vi "MCA_OpenDialog.vi"() -> (1 "要打开的数据文件路径： 2":path, 3 "是否取消？":bool)   [LabVIEW 2014]
panel:
  in  "取消":bool
  in  "确定":bool
  in  "要打开的数据文件路径：":path
  # "请选择要打开的数据文件的路径。能谱数据的格式为.tdms。"
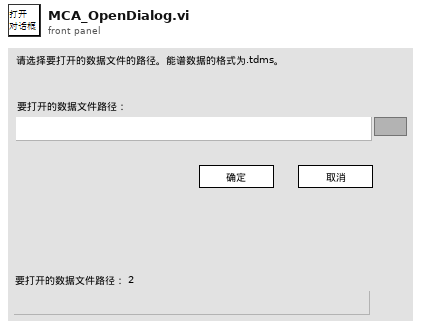
[diagram p1: front panel]
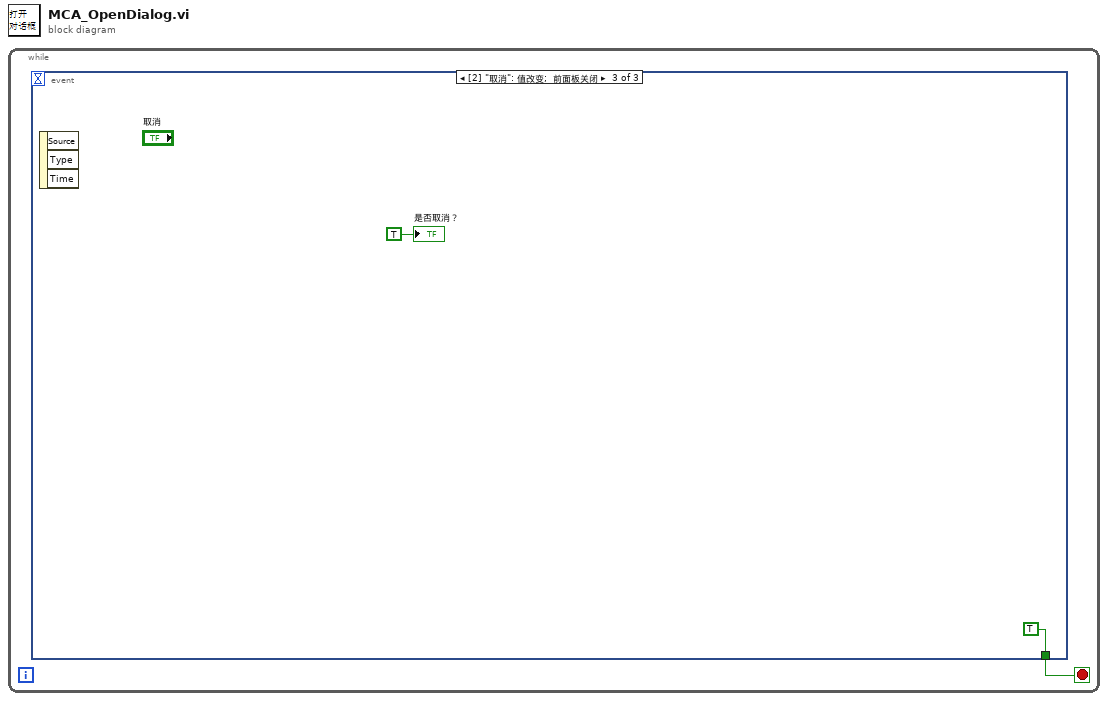
[diagram p0: block diagram]
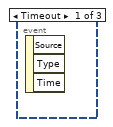
[diagram p2: hidden frame]
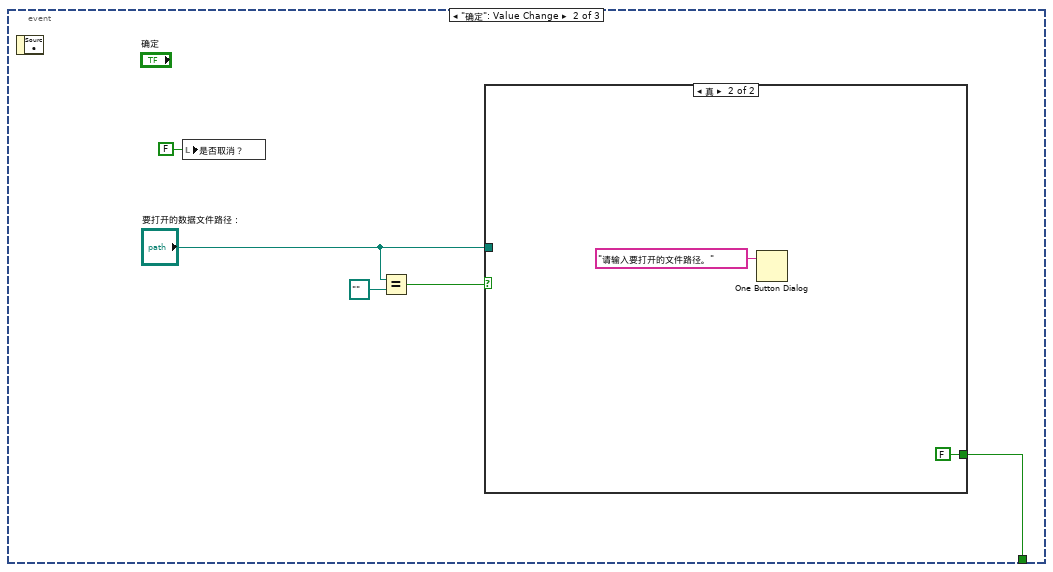
[diagram p3: hidden frame]
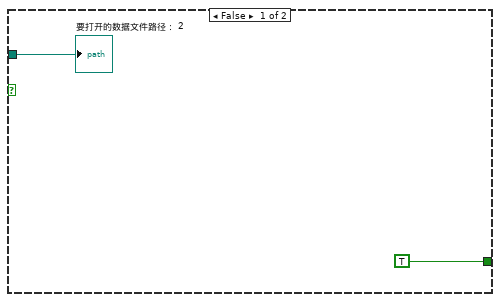
[diagram p4: hidden frame]
diagram:
  n1 = while {
    stop <- w1 stop-if-true
    n2 = event shown="[2] \"取消\": 值改变;  前面板关闭" {
      selector: _ -> [_ _ _]
      dyn-events: _ -> [_ _ _]
      timeout: _ -> [_ _ _]
      tunnel: [_ w2 TRUE] -> w1
      event Timeout {
        n3 = event-data() -> ()  [unwired: 1 in, 3 out]
      }
      event "确定": Value Change {
        n4 = event-data() -> ()  [unwired: 1 in, 1 out]
        n5 = local write "是否取消？"(FALSE ("是否取消？")) -> ()
        n6 = Equal?(x="要打开的数据文件路径：", y=path "") -> (x = y?=w3:bool)
        n7 = case shown="真" w3 {
          tunnel: "要打开的数据文件路径：" -> [w8 _]
          tunnel: [TRUE FALSE] -> w2
          frame False {
            "要打开的数据文件路径： 2" <- w8
          }
          frame True {
            n8 = One Button Dialog(message="请输入要打开的文件路径。" ("消息")) -> ()  [unwired: 1 in, 1 out]
          }
        }
      }
      event "取消": Value Change; Panel Close {
        n9 = event-data() -> ()  [unwired: 1 in, 3 out]
        "是否取消？" <- TRUE ("是否取消？")
      }
    }
  }
